vi "Adjust Frame Size.vi"(10 "Byte multiple (64)":i32=64, 11 "original size in":i32) -> (1 "size changed?":bool, 2 "adjusted size":i32, 3 "original size out":i32)   [LabVIEW 2020]
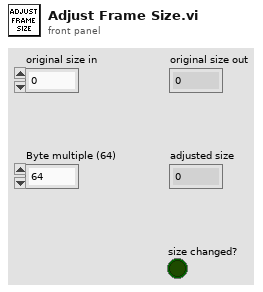
[diagram p1: front panel]
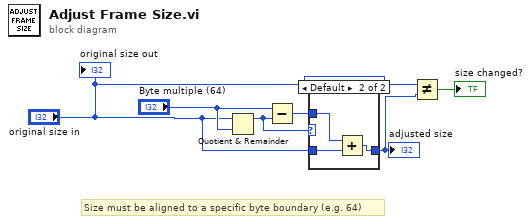
[diagram p0: block diagram]
diagram:
  # "Size must be aligned to a specific byte boundary (e.g. 64)"
  n1 = Quotient & Remainder(x="original size in", y="Byte multiple (64)") -> (x-y*floor(x/y)=w4:i32)  [unwired: 1 out]
  n2 = Subtract(x="Byte multiple (64)", y=w4) -> (x-y=w5:i32)
  n3 = case shown="Default" w4 {
    tunnel: w5 -> [_ w10]
    tunnel: "original size in" -> [w7 w9]
    tunnel: [w7 w8] -> w3
    frame 0 {
    }
    frame Default {
      n4 = Add(x=w10, y=w9) -> (x+y=w8:i32)
    }
  }
  "adjusted size" <- w3
  n5 = Not Equal?(x="original size in", y=w3) -> (x != y?=→"size changed?":bool)
  "original size out" <- "original size in"
